vi "determine_fourier_component.vi"(6 "baseline magnitude":dbl, 7 "baseline phase":dbl, 9 "RX frequency":dbl, 10 "phase":cluster{"f0":dbl, "df":dbl, "phase":dbl[]}, 11 "magnitude":cluster{"f0":dbl, "df":dbl, "magnitude":dbl[]}) -> (2 "RX phase":dbl, 3 "RX magnitude":dbl)   [LabVIEW 2019]
panel:
  in  "Use 3 points around RX frequ.":bool
  out "actual receive frequency":dbl
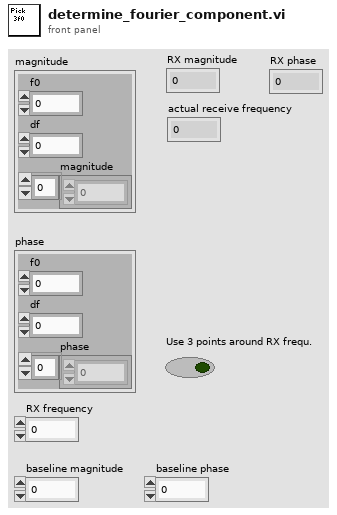
[diagram p1: front panel]
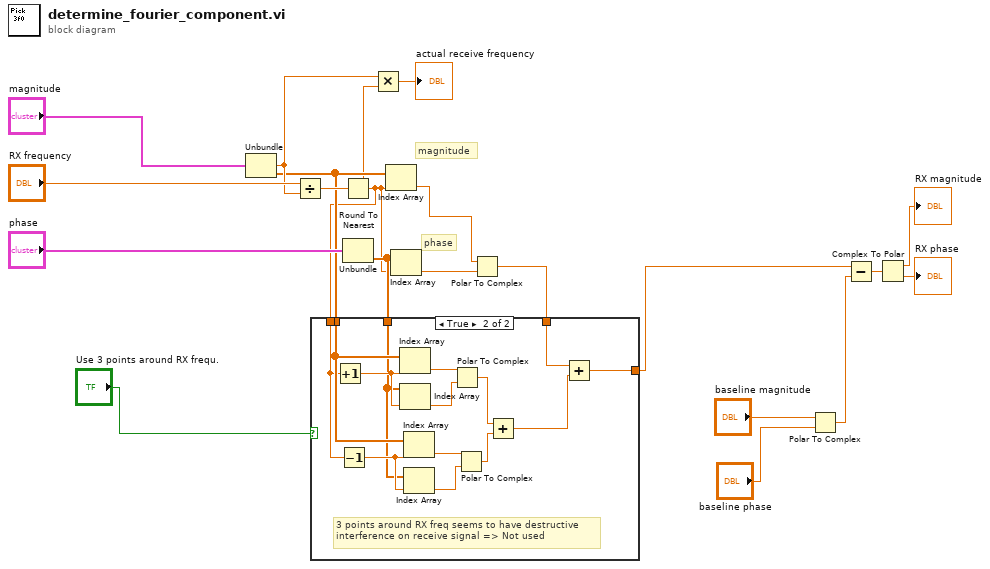
[diagram p0: block diagram]
diagram:
  # "phase"
  # "magnitude"
  n1 = Unbundle("magnitude") -> ("df"=w8:dbl, "magnitude"=w6:dbl[])  [unwired: 1 out]
  n2 = Divide(x="RX frequency", y=w8) -> (x/y=w11:dbl)
  n3 = Round To Nearest(number=w11) -> (nearest integer value=w4:dbl)
  n4 = Unbundle("phase") -> ("phase"=w5:dbl[])  [unwired: 2 out]
  n5 = Multiply(x=w8, y=w4) -> (x*y=→"actual receive frequency":dbl)
  n6 = Index Array(array=w6, index=w4) -> (element=w9:dbl)
  n7 = Index Array(array=w5, index=w4) -> (element=w15:dbl)
  n8 = Polar To Complex(1:w15, 2:w9) -> (0:w3:cdb)
  n9 = case shown="True" "Use 3 points around RX frequ." {
    tunnel: w6 -> [_ w29]
    tunnel: w5 -> [_ w28]
    tunnel: w4 -> [_ w27]
    tunnel: w3 -> [w21 w24]
    tunnel: [w21 w22] -> w2
    frame False {
    }
    frame True {
      # "3 points around RX freq seems to have destructive\ninterference on receive signal => Not used"
      n10 = Increment(x=w27) -> (x+1=w35:dbl)
      n11 = Decrement(x=w27) -> (x-1=w30:dbl)
      n12 = Index Array(array=w29, index=w35) -> (element=w34:dbl)
      n13 = Index Array(array=w28, index=w35) -> (element=w33:dbl)
      n14 = Index Array(array=w29, index=w30) -> (element=w31:dbl)
      n15 = Index Array(array=w28, index=w30) -> (element=w32:dbl)
      n16 = Polar To Complex(1:w33, 2:w34) -> (0:w25:cdb)
      n17 = Polar To Complex(1:w32, 2:w31) -> (0:w26:cdb)
      n18 = Add(x=w25, y=w26) -> (x+y=w23:cdb)
      n19 = Add(x=w24, y=w23) -> (x+y=w22:cdb)
    }
  }
  n20 = Polar To Complex(1:"baseline phase", 2:"baseline magnitude") -> (0:w18:cdb)
  n21 = Subtract(x=w2, y=w18) -> (x-y=w19:cdb)
  n22 = Complex To Polar(r * e^(i*theta)=w19) -> (r=→"RX magnitude":dbl, theta=→"RX phase":dbl)
